vi "Wash Options.vi"(8 "error in":errorcluster, 11 "input":T2) -> (0 "error out":errorcluster, 1 "output":T2, 3 "Array":T1[](array[typedef])=[enum."Under Body Wash", enum."Bug Remover", enum."Pre-soak", enum."High Pressure Wash", enum."Low Pressure Wash", enum."Spot Free Rinse", enum."Tire Shine Foam", enum."Air Dry"])   [LabVIEW 2024]
uses:
  ctl/Wash Options in.ctl
  ctl/WashOptionsTypedef.ctl
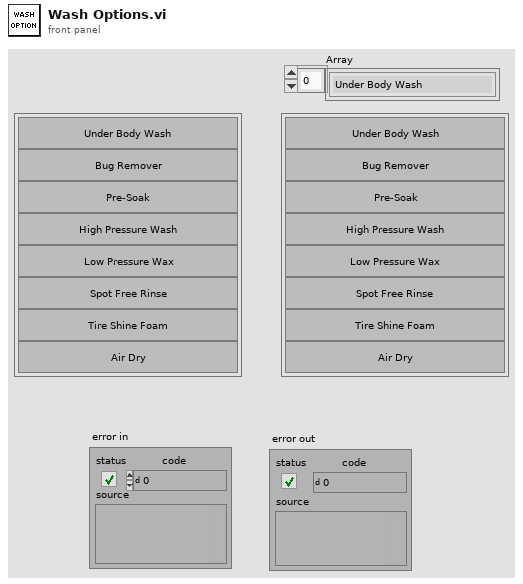
[diagram p1: front panel]
types:
  T1 = typedef "WashOptionsTypedef.ctl" = enum16{"Under Body Wash", "Bug Remover", "Pre-soak", "High Pressure Wash", "Low Pressure Wash", "Spot Free Rinse", "Tire Shine Foam", "Air Dry"}
  T2 = typedef "Wash Options in.ctl" = cluster{"Under Body Wash":bool, "Bug Remover":bool, "Pre-Soak":bool, "High Pressure Wash":bool, "Low Pressure Wax":bool, "Spot Free Rinse":bool, "Tire Shine Foam":bool, "Air Dry":bool}
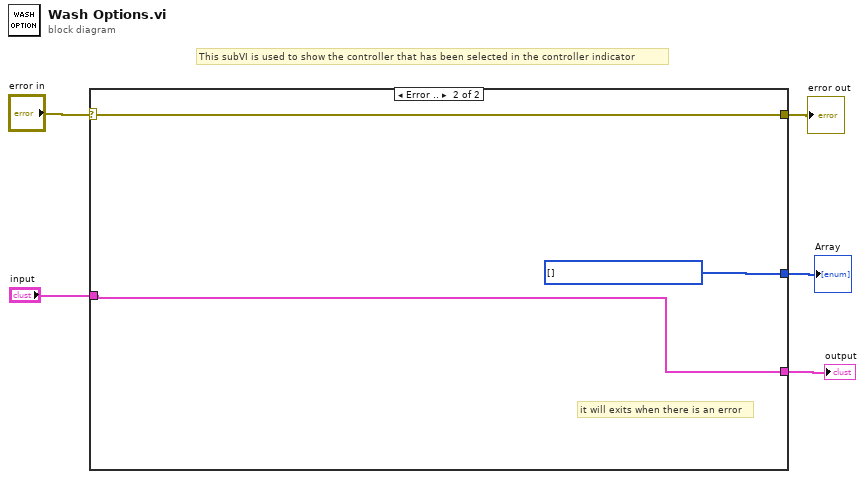
[diagram p0: block diagram]
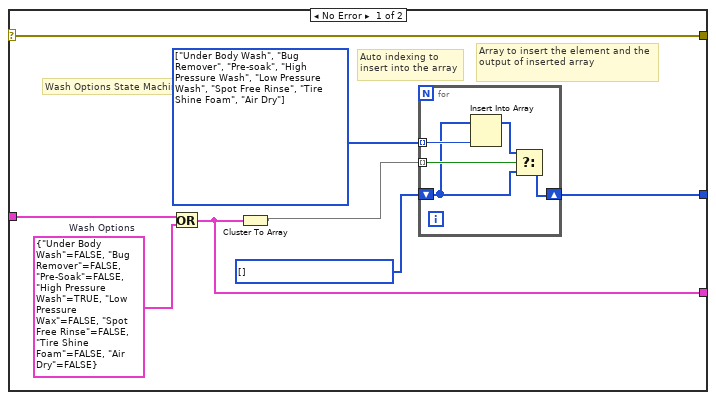
[diagram p2: hidden frame]
diagram:
  # "This subVI is used to show the controller that has been selected in the controller indicator"
  n1 = case shown="Error .." "error in" {
    selector: "error in" -> [w7 w19]
    tunnel: "input" -> [w12 w20]
    tunnel: [w9 w21] -> w1
    tunnel: [w8 w20] -> w5
    tunnel: [w7 w19] -> w2
    frame No Error {
      w11 = T2 {"Under Body Wash"=FALSE, "Bug Remover"=FALSE, "Pre-Soak"=FALSE, "High Pressure Wash"=TRUE, "Low Pressure Wax"=FALSE, "Spot Free Rinse"=FALSE, "Tire Shine Foam"=FALSE, "Air Dry"=FALSE}  # Wash Options
      w13 = T1[] [] items=["Under Body Wash", "Bug Remover", "Pre-soak", "High Pressure Wash", "Low Pressure Wash", "Spot Free Rinse", "Tire Shine Foam", "Air Dry"]
      w6 = T1[] [enum."Under Body Wash", enum."Bug Remover", enum."Pre-soak", enum."High Pressure Wash", enum."Low Pressure Wash", enum."Spot Free Rinse", enum."Tire Shine Foam", enum."Air Dry"] items=["Under Body Wash", "Bug Remover", "Pre-soak", "High Pressure Wash", "Low Pressure Wash", "Spot Free Rinse", "Tire Shine Foam", "Air Dry"]
      # "Array to insert the element and the output of inserted array"
      # "Auto indexing to insert into the array"
      # "Wash Options State Machine"
      n2 = Or(x=w12, y=w11) -> (x .or. y?=w8:T2)
      n3 = Cluster To Array(cluster=w8) -> (array=w10:bool[])
      n4 = for {
        tunnel: w6 -> [w17] mode=indexing
        shift-right: [w16] -> w9
        shift-left: w13 -> [w14]
        tunnel: w10 -> [w15] mode=indexing
        n5 = Insert Into Array "Insert Into Array"(array=w14, new element=w17) -> (w18:T1[])  [unwired: 1 in]
        n6 = Select(t=w18, s=w15, f=w14) -> (s? t:f=w16:T1[])
      }
    }
    frame Error {
      w21 = T1[] [] items=["Under Body Wash", "Bug Remover", "Pre-soak", "High Pressure Wash", "Low Pressure Wash", "Spot Free Rinse", "Tire Shine Foam", "Air Dry"]
      # "it will exits when there is an error"
    }
  }
  "output" <- w5
  "error out" <- w2
  "Array" <- w1
